vi "LUCS001RT_FIFO_WaitForCharacter.vi"(6 "stop":bool, 7 "timeout in ms (-1)":i32=1000, 8 "error in":errorcluster, 10 "Character":string, 11 "GPS Queue":refnum<queue>) -> (0 "error out":errorcluster, 2 "Character Out":string, 3 "GPS Queue DUP":refnum<queue>, 4 "TimedOut":bool)   [LabVIEW 2024]
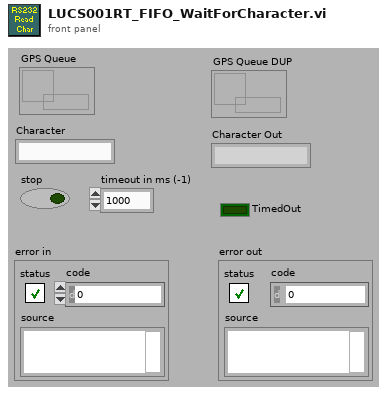
[diagram p1: front panel]
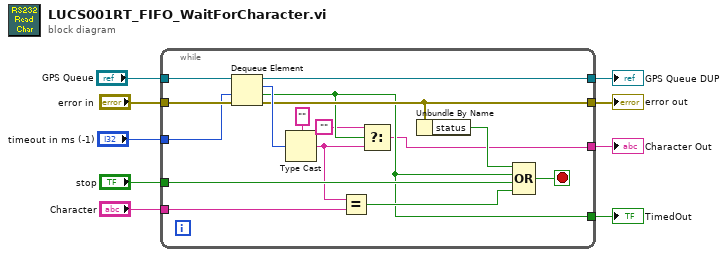
[diagram p0: block diagram]
diagram:
  n1 = while {
    tunnel: "error in" -> [w19]
    tunnel: [w15] -> w8
    tunnel: "stop" -> [w23]
    tunnel: "Character" -> [w22]
    tunnel: [w13] -> w5
    tunnel: [w11] -> w4
    tunnel: "GPS Queue" -> [w18]
    tunnel: [w16] -> w2
    tunnel: "timeout in ms (-1)" -> [w14]
    stop <- w25 stop-if-true
    n2 = Dequeue Element(queue=w18, timeout in ms (-1)=w14, error in (no error)=w19) -> (queue out=w16:refnum<queue>, element=w17:u8, timed out?=w13:bool, error out=w15:errorcluster)
    n3 = Type Cast(type="", x=w17) -> (*(type *) &x=w12:string)
    n4 = Equal?(x=w12, y=w22) -> (x = y?=w21:bool)
    n5 = Select(t="", s=w13, f=w12) -> (s? t:f=w11:string)
    n6 = Unbundle By Name(w15) -> ("status"=w24:bool)
    n7 = Compound Arithmetic op=OR(w24, w13, w23, w21) -> (w25:bool)
  }
  "error out" <- w8
  "TimedOut" <- w5
  "Character Out" <- w4
  "GPS Queue DUP" <- w2
